vi "Set Param.vi"(8 "error in":errorcluster, 10 "Data Cluster":T1 {"Actual_Data"."tТермошкаф, °С" format="%3.1f"; "Actual_Data"."tКД30, °С" format="%3.2f"; "Actual_Data"."m весы, г" format="%.4f"; "Actual_Data"."Vо2,\nсм3" format="%.4f"; "Actual_Data"."Кпрж2 Е-3,\nмкм2" format="%.4f"; "Actual_Data"."Vо1,\nсм3" format="%.2f град.С"; "Actual_Data"."Кпрж1 Е-3,\nмкм2" format="Р2 %#.2f МПа"; "Actual_Data"."Qо1,\nсм3/мин" format="Р2 %#.2f МПа"; "Actual_Data"."Рдм\nрасчётное,\nМПа" format="Р2 %#.2f МПа"; "appended array"."tТермошкаф, °С" format="%3.1f"; "appended array"."tКД30, °С" format="%3.2f"; "appended array"."m весы, г" format="%.4f"; "appended array"."Vо2,\nсм3" format="%.4f"; "appended array"."Кпрж2 Е-3,\nмкм2" format="%.4f"; "appended array"."Vо1,\nсм3" format="%.2f град.С"; "appended array"."Кпрж1 Е-3,\nмкм2" format="Р2 %#.2f МПа"}, 11 "Module ID":i32=-1) -> (0 "error out":errorcluster)   [LabVIEW 2018]
doc: "_____\nCreated using DQMH Event Scripter 6.1.0.128."
uses:
  Data Control.ctl
  Graph_data_collector.lvlib
  Module Data--cluster.ctl
  Set Param Argument--cluster.ctl
  Graph_UI.lvlib
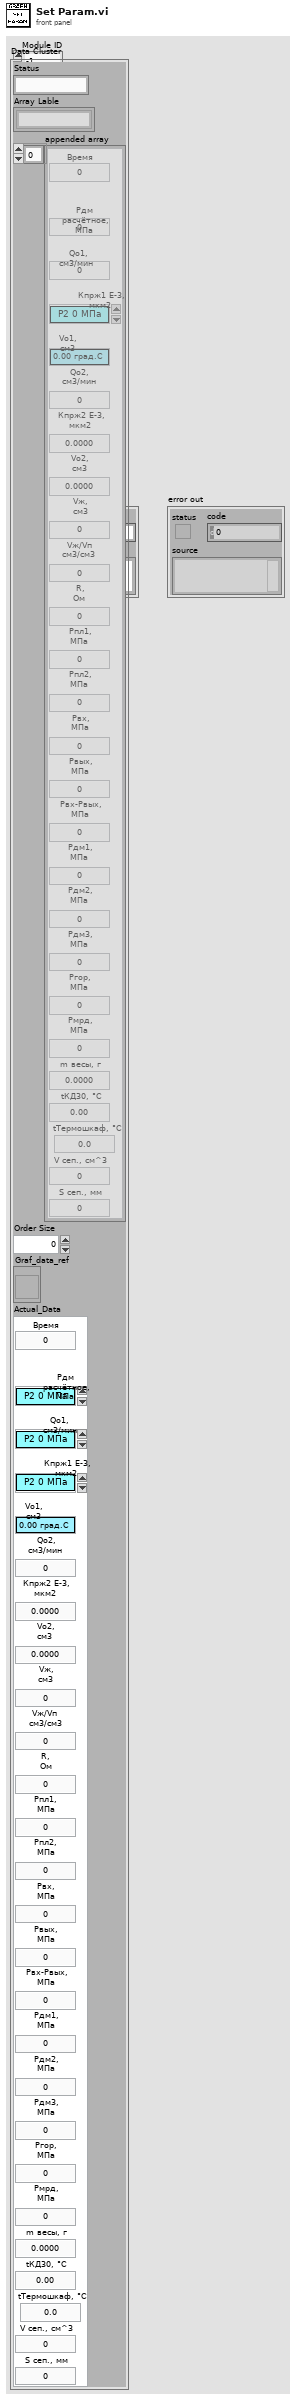
[diagram p1: front panel]
types:
  T1 = typedef "Graph_data_collector.lvlib/Module Data--cluster.ctl" = cluster{"Status":string, "Array Lable":string[], "appended array":T2[], "Order Size":u32, "Graf_data_ref":refnum<vi>, "Actual_Data":T2}
  T2 = typedef "Graph_data_collector.lvlib/Data Control.ctl" = cluster{"Время":dbl, "Рдм\nрасчётное,\nМПа":dbl, "Qо1,\nсм3/мин":dbl, "Кпрж1 Е-3,\nмкм2":dbl, "Vо1,\nсм3":dbl, "Qо2,\nсм3/мин":dbl, "Кпрж2 Е-3,\nмкм2":dbl, "Vо2,\nсм3":dbl, "Vж,\nсм3":dbl, "Vж/Vп\nсм3/см3":dbl, "R,\nОм":dbl, "Рпл1,\nМПа":dbl, "Рпл2,\nМПа":dbl, "Рвх,\nМПа":dbl, "Рвых,\nМПа":dbl, "Рвх-Рвых,\nМПа":dbl, "Рдм1,\nМПа":dbl, "Рдм2,\nМПа":dbl, "Рдм3,\nМПа":dbl, "Ргор,\nМПа":dbl, "Рмрд,\nМПа":dbl, "m весы, г":dbl, "tКД30, °С ":dbl, "tТермошкаф, °С":dbl, "V сеп., см^3 ":dbl, "S сеп., мм":dbl}
  T3 = typedef "Set Param Argument--cluster.ctl" = cluster{"Module ID":i32, "Data Cluster":T1}
  T4 = typedef "Graph_data_collector.lvlib/Graph_UI.lvlib/Request Events--cluster.ctl" = cluster{"Stop Module":refnum<user-event>, "Show Panel":refnum<user-event>, "Hide Panel":refnum<user-event>, "Show Diagram":refnum<user-event>, "Get Module Execution Status":refnum<user-event>, "New Data":refnum<user-event>, "SetP":refnum<user-event>}
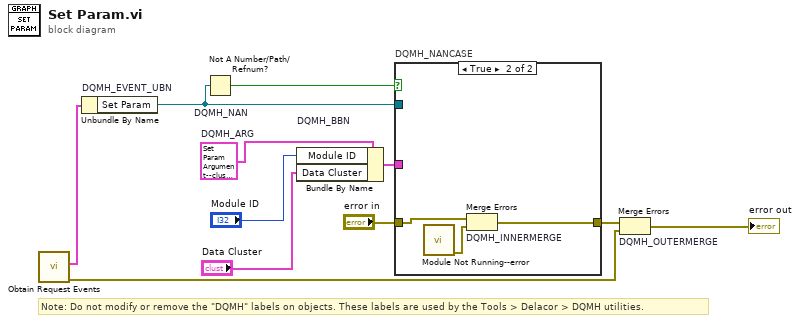
[diagram p0: block diagram]
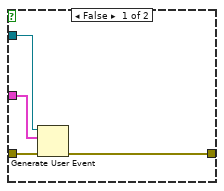
[diagram p2: hidden frame]
diagram:
  w5 = T3 {"Module ID"=-1, "Data Cluster"={"Status"="", "Array Lable"=[], "appended array"=[], "Order Size"=0, "Graf_data_ref"=refnum, "Actual_Data"={"Время"=0.0, "Рдм\nрасчётное,\nМПа"=0.0, "Qо1,\nсм3/мин"=0.0, "Кпрж1 Е-3,\nмкм2"=0.0, "Vо1,\nсм3"=0.0, "Qо2,\nсм3/мин"=0.0, "Кпрж2 Е-3,\nмкм2"=0.0, "Vо2,\nсм3"=0.0, "Vж,\nсм3"=0.0, "Vж/Vп\nсм3/см3"=0.0, "R,\nОм"=0.0, "Рпл1,\nМПа"=0.0, "Рпл2,\nМПа"=0.0, "Рвх,\nМПа"=0.0, "Рвых,\nМПа"=0.0, "Рвх-Рвых,\nМПа"=0.0, "Рдм1,\nМПа"=0.0, "Рдм2,\nМПа"=0.0, "Рдм3,\nМПа"=0.0, "Ргор,\nМПа"=0.0, "Рмрд,\nМПа"=0.0, "m весы, г"=0.0, "tКД30, °С "=0.0, "tТермошкаф, °С"=0.0, "V сеп., см^3 "=0.0, "S сеп., мм"=0.0}}}  # DQMH_ARG
  # "Note: Do not modify or remove the \"DQMH\" labels on objects. These labels are used by the Tools > Delacor > DQMH utilities."
  n1 = call "Obtain Request Events.vi"() -> ("error out"=w2:errorcluster, "Graph_UI Request Events"=w1:T4)  [unwired: 10 in]
  n2 = Unbundle By Name "DQMH_EVENT_UBN"(w1) -> ("Set Param"=w7:refnum<user-event>)
  n3 = Not A Number/Path/Refnum? "DQMH_NAN"(number/path/refnum=w7) -> (NaN/Path/Refnum?=w8:bool)
  n4 = Bundle By Name "DQMH_BBN"(cluster=w5, "Module ID"="Module ID", "Data Cluster"="Data Cluster") -> (w9:T3)
  n5 = case "DQMH_NANCASE" shown="True" w8 {
    tunnel: "error in" -> [w15 w18]
    tunnel: [w14 w17] -> w6
    tunnel: w7 -> [w13 _]
    tunnel: w9 -> [w12 _]
    frame False {
      n6 = Generate User Event(user event=w13, event data cluster=w12, error in=w15) -> (error out=w14:errorcluster)  [unwired: 1 in, 1 out]
    }
    frame True {
      n7 = call "Module Not Running--error.vi"() -> ("error out"=w16:errorcluster)  [unwired: 11 in]
      n8 = Merge Errors "DQMH_INNERMERGE"(w18, w16) -> (w17:errorcluster)
    }
  }
  n9 = Merge Errors "DQMH_OUTERMERGE"(w6, w2) -> (→"error out":errorcluster)
